vi "ScheduledCmdWindow.vi"(7 "Name (\"\" to Use UUID)":string="Event CSM") -> ()   [LabVIEW 2020, in "CSM-ScheduledCmdWindow.lvlib"]
uses:
  CSM-ScheduledCmdWindow.lvlib
  _support/Command Timer Item.ctl
  <userlib>/_Hooovahh/Array VIMs/Controls/Enum - Order Ascending Descending.ctl
  54d86923-07a1-4d7a-a70d-45b0863b869b.vi
  fe2ecfb7-eb08-4f89-820d-2b95152fbf7e.vi
  dd2ac68a-60a3-4251-9735-56811cc0631c.vi
  96b01cc3-4e05-4812-bc78-c919a57353e8.vi
  <userlib>/_NEVSTOP/Communicable State Machine(CSM)/_Support/GlobalEvent/GEvt-Generate with Rule Check.vi
  <userlib>/_NEVSTOP/Communicable State Machine(CSM)/_Support/GlobalEvent/Cache-GEvt Refs.vi
  <userlib>/_NEVSTOP/Communicable State Machine(CSM)/AdvanceAPI/CSM - Revert Arguments-Safe String.vi
  <userlib>/_NEVSTOP/Communicable State Machine(CSM)/_Shared/Trim Single-line Text.vi
  <userlib>/_NEVSTOP/Communicable State Machine(CSM)/AdvanceAPI/CSM - Make String Arguments Safe.vi
  <userlib>/_NEVSTOP/Communicable State Machine(CSM)/AdvanceAPI/CSM - Break Down Multiple States String.vi
  <userlib>/_NEVSTOP/Communicable State Machine(CSM)/_Support/ChangeFlag/FlagInstance-GEvt Refs.vi
  <userlib>/_NEVSTOP/Communicable State Machine(CSM)/AdvanceAPI/CSM - Keywords.vi
  <userlib>/_NEVSTOP/Communicable State Machine(CSM)/_Support/ChangeFlag/ChangeFlag-Read.vi
  <userlib>/_NEVSTOP/Communicable State Machine(CSM)/AdvanceAPI/CSM - List Modules.vi
  <userlib>/_NEVSTOP/Communicable State Machine(CSM)/_Support/ChangeFlag/ChangeFlagDB.vi
  <userlib>/_NEVSTOP/Communicable State Machine(CSM)/_Support/GlobalEvent/FGV-GlobalEventRef(lvlibp).vi
  <userlib>/_NEVSTOP/Communicable State Machine(CSM)/_Support/GlobalEvent/FGV-GlobalEventQueues(lvlibp).vi
  <userlib>/_NEVSTOP/Communicable State Machine(CSM)/_Support/GlobalEvent/GEvt-Valid Subscribers.vi
  <userlib>/_NEVSTOP/Communicable State Machine(CSM)/_Support/GlobalEvent/LogFilter/LogFilter - Check.vi
  <userlib>/NEVSTOP-Programming-Palette/Dialog & Interface/_support/Autosize All MultiListbox Columns (Uniform Text)_nevstop.vi
  <userlib>/NEVSTOP-Programming-Palette/Dialog & Interface/Fit VI window to Largest Dec_nevstop.vi
  _support/Select Timestamp Dialog.vi
  <userlib>/NEVSTOP-Programming-Palette/Dialog & Interface/Fit VI window to Caller Center_nevstop.vi
  <userlib>/_NEVSTOP/Communicable State Machine(CSM)/addons/API-String-Arugments-Support/_Support/Data To API String Arguments.vi
  <userlib>/_NEVSTOP/Communicable State Machine(CSM)/_Polymophic/Add State(s) to Queue By BOOL(Element).vi
  <userlib>/_NEVSTOP/Communicable State Machine(CSM)/addons/API-String-Arugments-Support/_Support/Convert API String Arguments to Data(variant).vi
  <userlib>/_NEVSTOP/Communicable State Machine(CSM)/_Support/GlobalEvent/LogFilter/LogFilter.lvclass
  <userlib>/_NEVSTOP/Communicable State Machine(CSM)/Communicable State Machine.lvlib
panel:
  out "SharedData":T1[](array[typedef])
  in  "Multicolumn Listbox":i32[](listbox) caption="Table Control"
  in  "Remove Btn":bool
  in  "Add Btn":bool
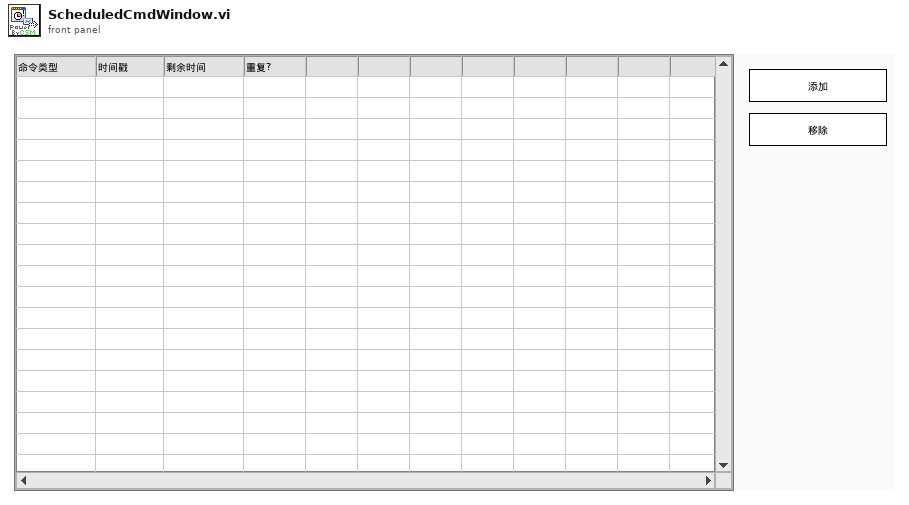
[diagram p1: front panel]
types:
  T1 = typedef "CSM-ScheduledCmdWindow.lvlib/Command Timer Item.ctl" = cluster{"Command":string, "TimeStamp":timestamp, "Daily?":bool}
  T2 = enum32{"Invalid", "Standard", "Closed", "Hidden", "Minimized", "Maximized"}
  T3 = enum32{"invalid app kind", "Development System", "Run Time System", "Student Edition", "Embedded LabVIEW", "Evaluation", "Custom"}
  T4 = typedef "Enum - Order Ascending Descending.ctl" = enum16{"Ascending", "Descending"}
  T5 = typedef "Communicable State Machine.lvlib/_CSM_Response Source Message.ctl" = cluster{"‘State":string, "’Arguments":string, "’Error":errorcluster}
  T6 = cluster{"Current VI Reference":refnum<vi>, "Close Panel on Exit?":bool}
  T7 = cluster{"Core":cluster{"Current VI Reference":refnum<vi>, "Close Panel on Exit?":bool}, "Your Boolean data":bool, "Your string data":string}
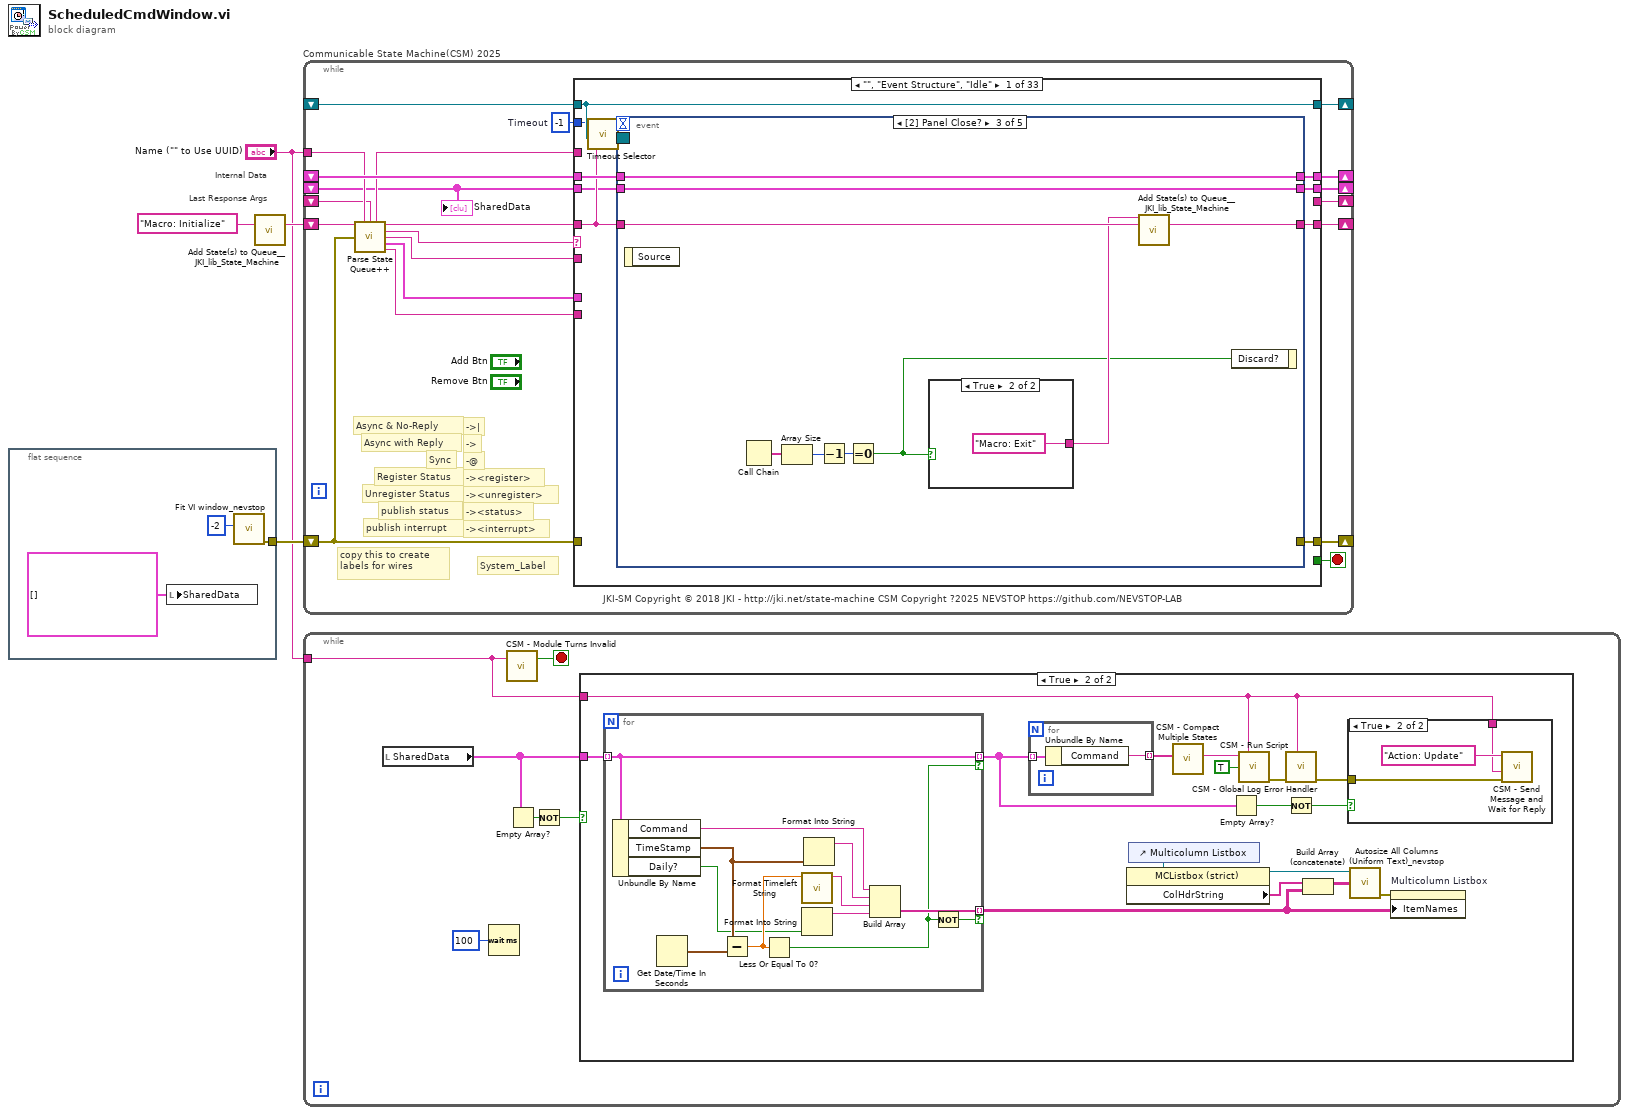
[diagram p0: block diagram]
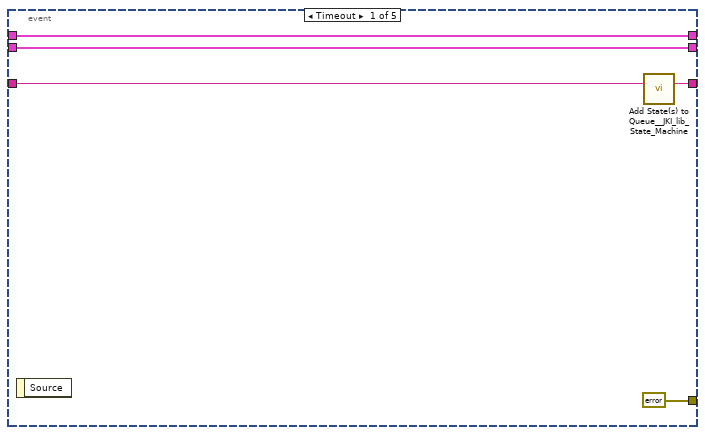
[diagram p2: hidden frame]
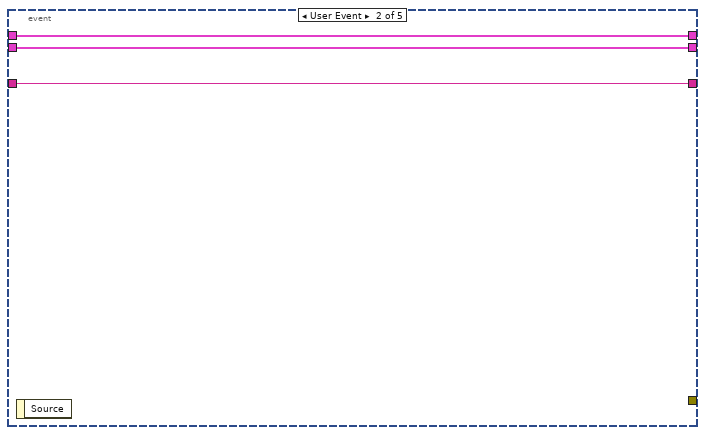
[diagram p3: hidden frame]
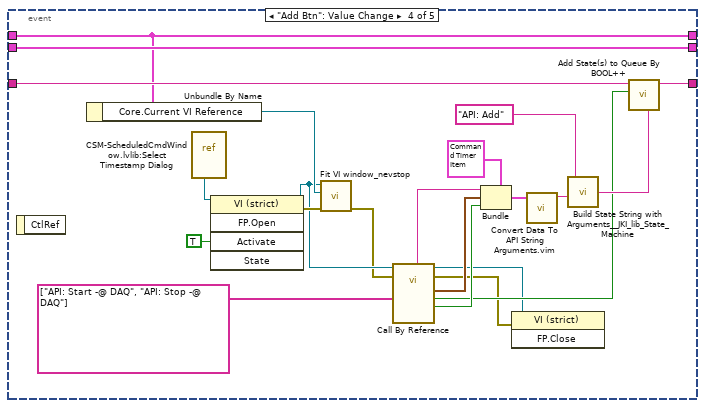
[diagram p5: hidden frame]
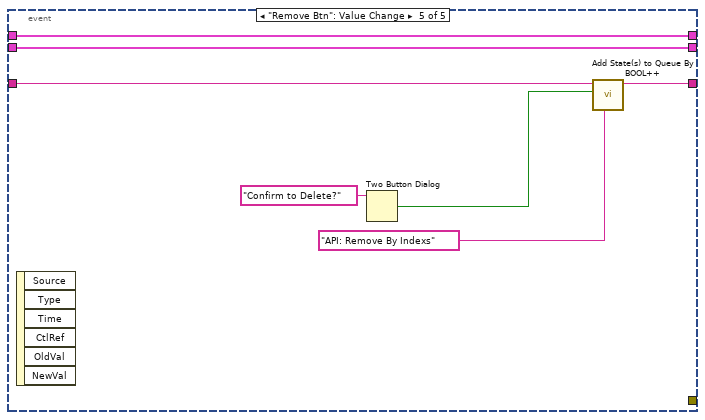
[diagram p6: hidden frame]
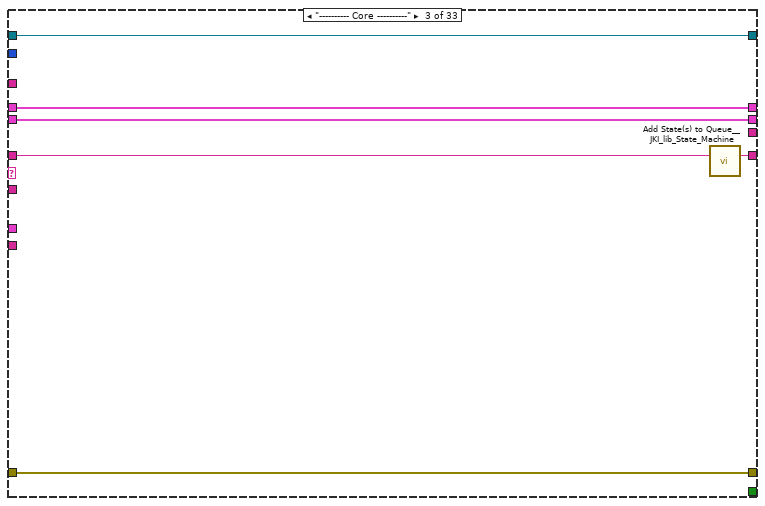
[diagram p8: hidden frame]
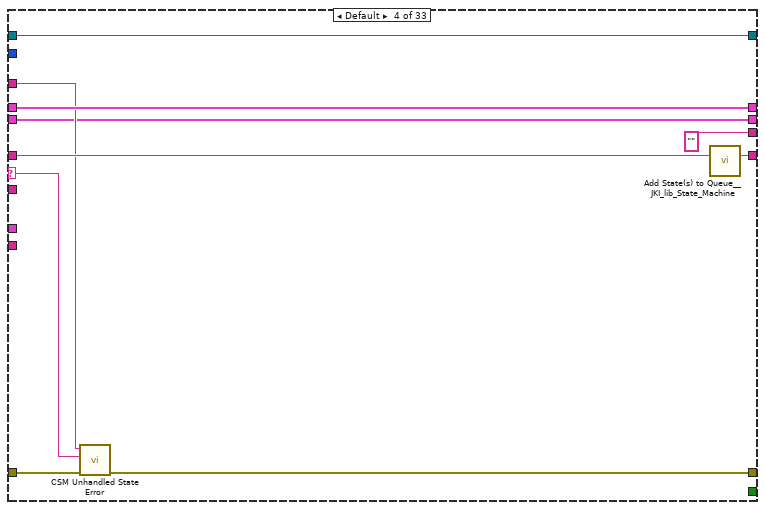
[diagram p9: hidden frame]
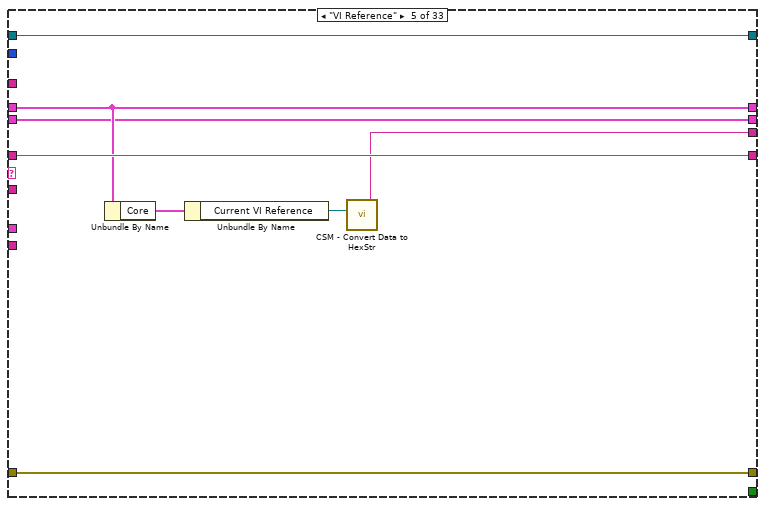
[diagram p10: hidden frame]
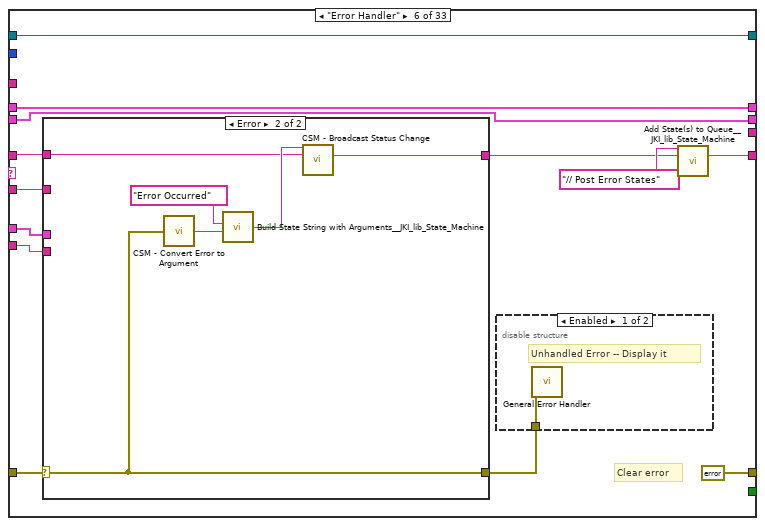
[diagram p11: hidden frame]
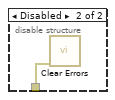
[diagram p12: hidden frame]
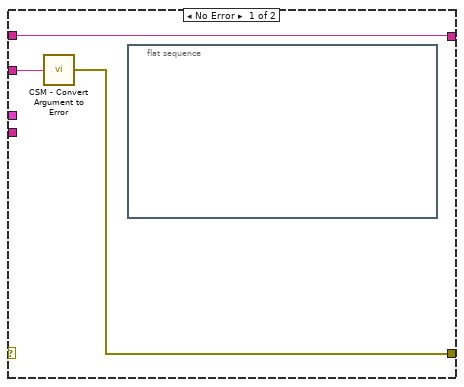
[diagram p13: hidden frame]
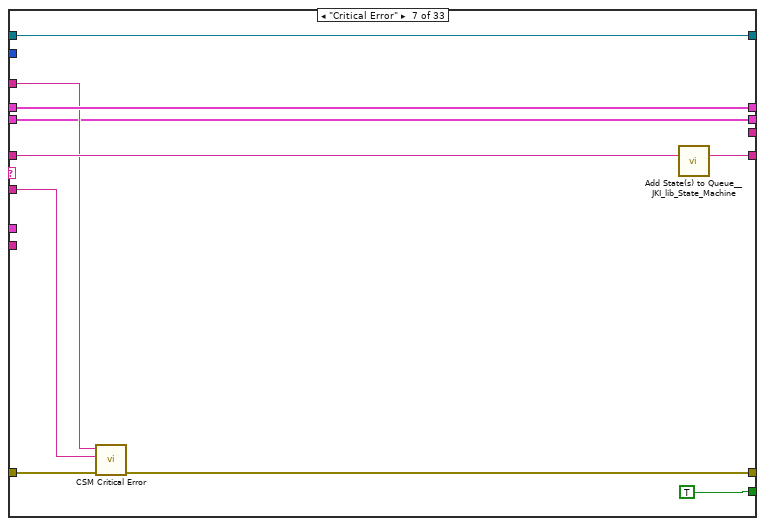
[diagram p14: hidden frame]
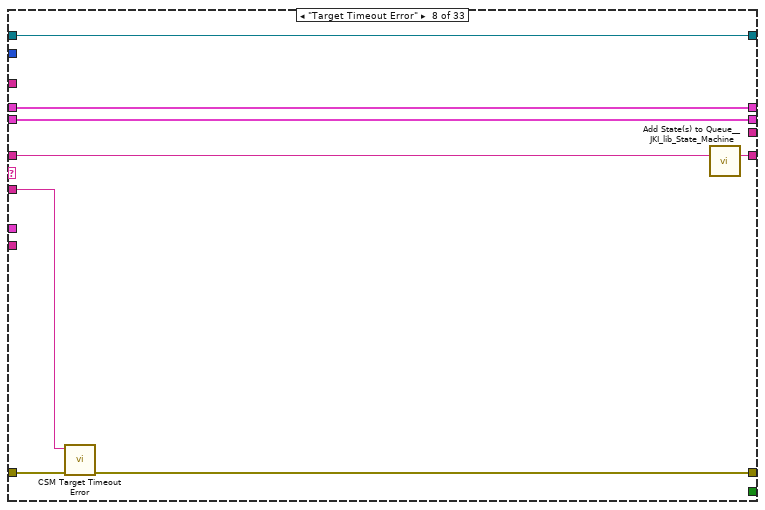
[diagram p15: hidden frame]
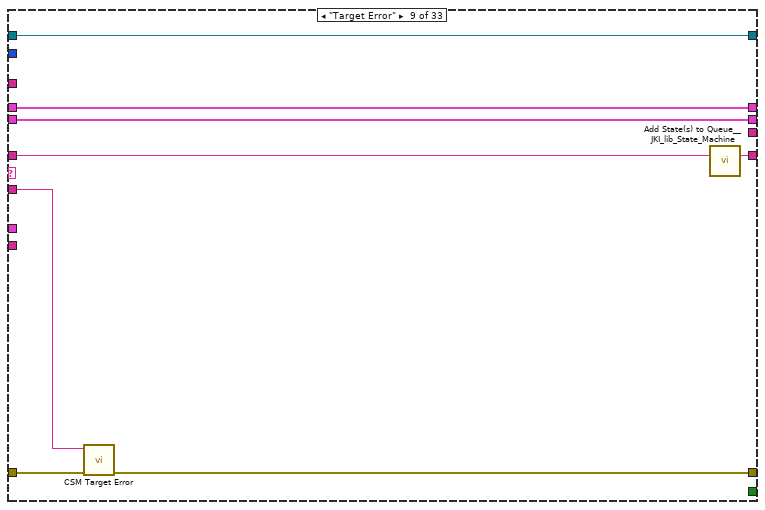
[diagram p16: hidden frame]
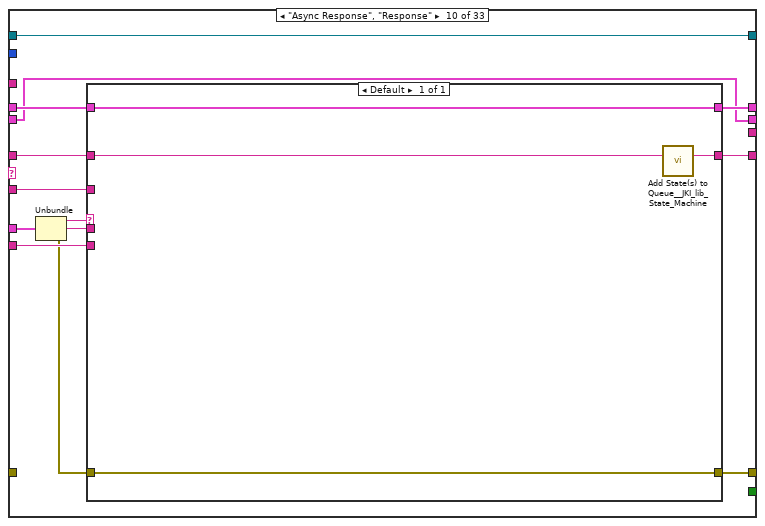
[diagram p17: hidden frame]
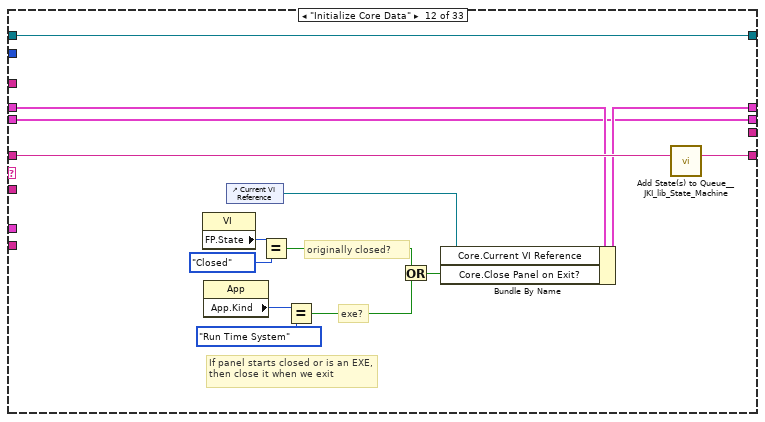
[diagram p19: hidden frame]
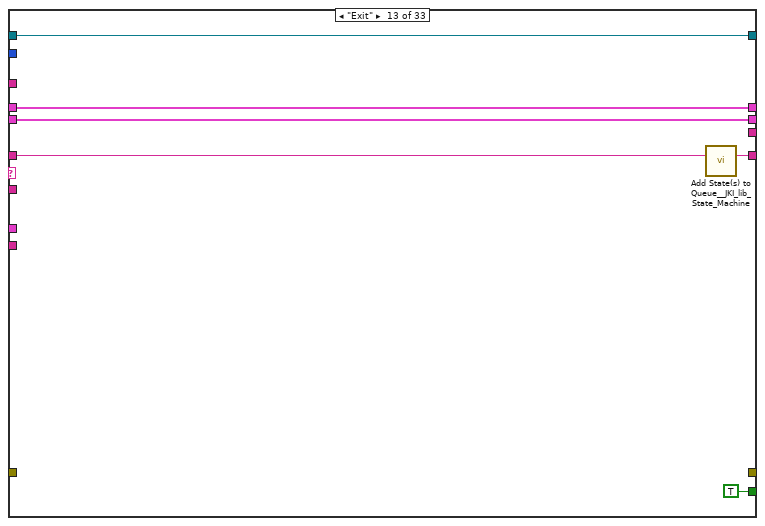
[diagram p20: hidden frame]
diagram:
  # "Last Response Args"
  # "Internal Data"
  n1 = flat-sequence {
    tunnel: [w6] -> w2
    frame #0 {
      n2 = local write "SharedData"(T1[] [] ("SharedData")) -> ()
      n3 = call-poly <userlib>:"Fit VI window_nevstop.vi"("border spacing (2 px)"=-2) -> ("error out"=w6:errorcluster)  [unwired: 5 in, 1 out]
    }
  }
  n4 = call <vilib>:"Add State(s) to Queue__JKI_lib_State_Machine.vi"("State(s) in (\"\")"="Macro: Initialize" ("Init State(\"Macro: Initialize\")")) -> ("States Out"=w3:string)  [unwired: 14 in]
  n5 = while "Communicable State Machine(CSM) 2025" {
    shift-right: [w23] -> _
    shift-left: _ -> [w22]
    shift-right: [w26] -> _
    shift-left: w2 -> [w20]
    shift-right: [w25] -> _
    shift-left: w3 -> [w27]
    tunnel: "Name (\"\" to Use UUID)" -> [w16]
    shift-right: [w19] -> _
    shift-left: _ -> [w11]
    shift-right: [w18] -> _
    shift-left: _ -> [w17]
    shift-right: [w9] -> _
    shift-left: _ -> [w8]
    stop <- w24 stop-if-true
    w21 = -1  # Timeout
    # "-><interrupt>"
    # "-><status>"
    # "-><unregister>"
    # "-><register>"
    # "-@"
    # "->"
    # "->|"
    # "publish interrupt"
    # "publish status"
    # "Unregister Status"
    # "Register Status"
    # "Sync"
    # "Async with Reply"
    # "Async & No-Reply"
    # "copy this to create labels for wires"
    # "System_Label"
    # "JKI-SM Copyright © 2018 JKI - http://jki.net/state-machine CSM Copyright ?2025 NEVSTOP https://github.com/NEVSTOP-LAB"
    n6 = call <userlib>:"Parse State Queue++.vi"("State Queue"=w27, "Name (\"\" to Use UUID)"=w16, "Response Arguments"=w11, "Previous Error"=w20) -> ("Name Used"=w12:string, "Remaining States"=w28:string, "Current State"=w15:string, "Arguments"=w10:string, "Additional Information"=w14:T5, "Source CSM"=w13:string)  [unwired: 6 in]
    n7 = case shown="\"\", \"Event Structure\", \"Idle\"" w15 {
      selector: w15 -> [_ _ _ w99 _ _ _ _ _ _ _ _ _ _ _ _ _ _ _ _ _ _ _ _ _ _ _ _ _ _ _ _ _]
      tunnel: w28 -> [w31 w89 w95 w105 w112 w119 w146 w155 w163 w174 w184 w198 w204 w209 w217 w221 w229 w234 w242 w247 w252 w263 w270 w282 w347 w353 w365 w369 w380 w393 w401 w408 w429]
      tunnel: w10 -> [_ _ _ _ _ w117 w142 w150 w159 w168 _ _ _ _ _ _ _ _ _ _ _ _ w266 w277 _ _ _ _ w373 w386 _ _ _]
      tunnel: w22 -> [w37 w88 w92 w103 w111 w125 w147 w153 w161 w172 w183 w192 w202 w207 _ w220 w225 w232 w241 w246 w250 w261 w268 w279 w345 w351 w363 w368 w379 w392 w399 w406 w427]
      tunnel: [w36 _ w93 w97 w113 errorcluster {"status"=FALSE, "code"=0, "source"=""} ("error out") w139 w149 w157 w171 _ _ _ _ _ w222 w226 _ w236 w245 _ _ w267 w280 _ _ _ _ w371 w383 _ _ _] -> w26
      tunnel: w20 -> [_ _ w93 w98 w113 w123 w140 w151 w158 _ _ _ _ _ _ w222 _ _ _ _ _ _ _ _ _ _ _ _ _ _ _ _ _]
      tunnel: [w38 w89 w94 w104 w112 w121 w145 w154 w162 w175 w184 w197 w203 w208 w216 w221 w228 w233 w242 w247 w251 w262 w269 w281 w346 w352 w364 w369 w380 w393 w400 w407 w428] -> w25
      tunnel: [_ _ _ _ _ _ TRUE _ _ _ _ _ TRUE _ _ _ _ _ _ _ _ _ _ _ _ _ _ _ _ _ _ _ _] -> w24
      tunnel: [w35 w88 w92 w103 w111 w125 w147 w153 w161 w173 w183 w196 w202 w207 w215 w220 w225 w232 w241 w246 w250 w261 w268 w279 w345 w351 w363 w368 w379 w392 w399 w406 w427] -> w23
      tunnel: w21 -> [w33 _ _ _ _ _ _ _ _ _ _ _ _ _ _ _ _ _ _ _ _ _ _ _ _ _ _ _ _ _ _ _ _]
      tunnel: w13 -> [_ _ _ _ _ w116 _ _ _ w169 _ _ _ _ _ _ _ _ _ _ _ _ _ _ _ _ _ _ _ _ _ _ _]
      tunnel: w14 -> [_ _ _ _ _ w115 _ _ _ w170 _ _ _ _ _ _ _ _ _ _ _ _ _ _ _ _ _ _ _ _ _ _ _]
      tunnel: [_ _ _ "" w107 _ _ _ _ _ _ _ _ _ _ _ _ _ _ _ _ _ _ _ _ _ _ _ _ _ _ _ _] -> w19
      tunnel: [w34 w87 w91 w101 w110 w124 w143 w152 w160 w176 w182 w186 w200 w206 w211 w219 w224 w231 w240 w244 w249 w260 w265 w276 w344 w349 w356 w367 w378 w391 w398 w405 w426] -> w18
      tunnel: w17 -> [w34 w87 w91 w101 w110 w124 w143 w152 w160 w176 w182 w186 w200 w206 w211 w219 w224 w231 _ w244 w249 w260 w265 w276 w344 w349 w356 w367 w378 w391 w398 w405 w426]
      tunnel: w12 -> [_ _ _ w100 _ _ w141 _ _ _ _ _ _ _ _ _ _ _ w239 _ _ _ _ _ _ _ _ _ _ _ _ _ _]
      tunnel: [w29 w86 w90 w96 w106 w114 w138 w148 w156 w164 w181 w185 w199 w205 T1[] [] w218 w223 w230 w235 w243 w248 w259 w264 w275 w343 w348 w354 w366 w375 w389 w397 w402 w425] -> w9
      tunnel: w8 -> [w30 w86 w90 w96 w106 w114 w138 w148 w156 w164 w181 w185 w199 w205 _ w218 w223 w230 w235 w243 w248 w259 w264 w275 w343 w348 w354 w366 w376 w390 w397 w404 w425]
      frame "", "Event Structure", "Idle" {
        n8 = call <userlib>:"Timeout Selector.vi"("Remaining States"=w31, "Timeout Expected"=w33) -> ("Timeout"=w32:i32)  [unwired: 5 in]
        n9 = event shown="[2] Panel Close?" {
          selector: w34 -> [_ _ _ _ _]
          dyn-events: _ -> [_ _ _ _ _]
          timeout: w32 -> [_ _ _ _ _]
          tunnel: w31 -> [w43 w45 w55 w72 w82]
          tunnel: [w42 w45 w54 w73 w83] -> w38
          tunnel: w37 -> [w41 w46 w53 w68 w85]
          tunnel: [errorcluster {"status"=FALSE, "code"=0, "source"=""} ("error out") _ _ _ _] -> w36
          tunnel: [w41 w46 w53 w68 w85] -> w35
          tunnel: w30 -> [w39 w44 w52 w78 w84]
          tunnel: [w39 w44 w52 w78 w84] -> w29
          event Timeout {
            n10 = event-data() -> ()  [unwired: 1 in, 1 out]
            n11 = call <vilib>:"Add State(s) to Queue__JKI_lib_State_Machine.vi"("State(s) in (\"\")"=w43) -> ("States Out"=w42:string)  [unwired: 14 in]
          }
          event User Event {
            n12 = event-data() -> ()  [unwired: 1 in, 1 out]
          }
          event Panel Close? {
            n13 = event-data() -> ()  [unwired: 1 in, 1 out]
            n14 = Call Chain() -> (call chain=w47:string[])
            n15 = Array Size(array=w47) -> (size(s)=w48:i32)
            n16 = Decrement(x=w48) -> (x-1=w49:i32)
            n17 = Equal To 0?(x=w49) -> (x = 0?=w50:bool)
            n18 = case shown="True" w50 {
              tunnel: [_ "Macro: Exit"] -> w51
              frame False {
              }
              frame True {
              }
            }
            n19 = call <vilib>:"Add State(s) to Queue__JKI_lib_State_Machine.vi"("State(s) in Front (\"\")"=w51, "State(s) in (\"\")"=w55) -> ("States Out"=w54:string)  [unwired: 13 in]
            n20 = event-data("Discard?"=w50) -> ()  [unwired: 1 in, 1 out]
          }
          event "Add Btn": Value Change {
            n21 = event-data() -> ()  [unwired: 1 in, 1 out]
            n22 = Unbundle By Name(w68) -> ("Core.Current VI Reference"=w67:refnum<vi>)
            n23 = vi-ref "CSM-ScheduledCmdWindow.lvlib:Select Timestamp Dialog.vi"() -> (w70:refnum<vi>)
            n24 = invoke class="VI (strict)" method="FP.Open"(reference=w70, "Activate"=TRUE ("Activate?")) -> (reference out=w66:refnum<vi>, error out=w69:errorcluster)  [unwired: 3 in, 3 out]
            n25 = call-poly <userlib>:"Fit VI window_nevstop.vi"("Error In"=w69, "Background VI Ref (Callee's Caller)"=w67, "VI Ref (calling VI)"=w66) -> ("Error Out"=w60:errorcluster)  [unwired: 3 in, 1 out]
            n26 = call-by-ref "?"(reference=w66, error in=w60, "Command List"=string[] ["API: Start -@ DAQ", "API: Stop -@ DAQ"]) -> (reference out=w58:refnum<vi>, error out=w57:errorcluster, "Daily?"=w64:bool, "Cancelled?"=w63:bool, "Time Stamp out"=w61:timestamp, "Command out"=w62:string)  [unwired: 6 in, 1 out]
            n27 = Bundle(cluster=T1 {"Command"="", "TimeStamp"=timestamp(0 s since 1904-01-01), "Daily?"=FALSE} ("Cluster"), "Command"=w62, "TimeStamp"=w61, "Daily?"=w64) -> (w76:T1)
            n28 = invoke class="VI (strict)" method="FP.Close"(reference=w58, error in=w57) -> ()  [unwired: 1 in, 3 out]
            n29 = call "Convert Data To API String Arguments.vim"("Data"=w76) -> ("API String"=w75:string)  [unwired: 7 in, 1 out]
            n30 = call <vilib>:"Build State String with Arguments__JKI_lib_State_Machine.vi"("Arguments (\"\")"=w75, "State"="API: Add") -> ("State with Arguments"=w71:string)  [unwired: 4 in]
            n31 = call-poly <userlib>:"Add State(s) to Queue By BOOL++.vi"("FALSE (\"\")"=w71, "Condition"=w63, "State Queue (\"\")"=w72) -> ("Remaining States"=w73:string)  [unwired: 8 in]
          }
          event "Remove Btn": Value Change {
            n32 = event-data() -> ()  [unwired: 1 in, 6 out]
            n33 = Two Button Dialog(message="Confirm to Delete?") -> (T button?=w80:bool)  [unwired: 2 in]
            n34 = call-poly <userlib>:"Add State(s) to Queue By BOOL++.vi"("TRUE (\"\")"="API: Remove By Indexs" ("TRUE (\"\")"), "Condition"=w80, "State Queue (\"\")"=w82) -> ("Remaining States"=w83:string)  [unwired: 8 in]
          }
        }
      }
      frame "CSM Documentation" {
      }
      frame "---------- Core ----------" {
        n35 = call <vilib>:"Add State(s) to Queue__JKI_lib_State_Machine.vi"("State(s) in (\"\")"=w95) -> ("States Out"=w94:string)  [unwired: 14 in]
      }
      frame Default {
        n36 = call <userlib>:"CSM Unhandled State Error.vi"("error in (no error)"=w98, "Undefined State"=w99, "CSM Name"=w100) -> ("error out"=w97:errorcluster)  [unwired: 8 in]
        n37 = call <vilib>:"Add State(s) to Queue__JKI_lib_State_Machine.vi"("State(s) in (\"\")"=w105) -> ("States Out"=w104:string)  [unwired: 14 in]
      }
      frame "VI Reference" {
        n38 = Unbundle By Name(w111) -> ("Core"=w109:T6)
        n39 = Unbundle By Name(w109) -> ("Current VI Reference"=w108:refnum<vi>)
        n40 = call <userlib>:"CSM - Convert Data to HexStr.vi"("Variant"=w108) -> ("HEX String (0-9,A-F)"=w107:string)  [unwired: 8 in]
      }
      frame "Error Handler" {
        # "Clear error"
        n41 = case shown="Error" w123 {
          selector: w123 -> [_ w132]
          tunnel: [w130 w134] -> w120
          tunnel: w119 -> [w130 w133]
          tunnel: [w129 w132] -> w118
          tunnel: w117 -> [w131 _]
          tunnel: w116 -> [_ _]
          tunnel: w115 -> [_ _]
          frame No Error {
            n42 = call <userlib>:"CSM - Convert Argument to Error.vi"("Argument"=w131) -> ("Error"=w129:errorcluster)  [unwired: 4 in]
            n43 = flat-sequence {
              frame #0 {
              }
            }
          }
          frame Error {
            n44 = call <userlib>:"CSM - Convert Error to Argument.vi"("Error"=w132) -> ("Argument"=w136:string)  [unwired: 4 in]
            n45 = call <vilib>:"Build State String with Arguments__JKI_lib_State_Machine.vi"("Arguments (\"\")"=w136, "State"="Error Occurred" ("Status with Arguments")) -> ("State with Arguments"=w135:string)  [unwired: 4 in]
            n46 = call <userlib>:"CSM - Broadcast Status Change.vi"("Status With Arguments"=w135, "State Queue"=w133) -> ("Remaining States"=w134:string)  [unwired: 13 in]
          }
        }
        n47 = disable-structure shown="Enabled" {
          disable-tunnel: w118 -> [w127 w128]
          frame Enabled {
            # "Unhandled Error -- Display it"
            n48 = call <vilib>:"General Error Handler.vi"("error in (no error)"=w127) -> ()  [unwired: 10 in, 5 out]
          }
          frame Disabled {
            n49 = call <vilib>:"Clear Errors.vi"("error in (no error)"=w128) -> ()  [unwired: 5 in, 2 out]
          }
        }
        n50 = call <vilib>:"Add State(s) to Queue__JKI_lib_State_Machine.vi"("State(s) in Front (\"\")"="// Post Error States", "State(s) in (\"\")"=w120) -> ("States Out"=w121:string)  [unwired: 13 in]
      }
      frame "Critical Error" {
        n51 = call <userlib>:"CSM Critical Error.vi"("error in (no error)"=w140, "Arugments (As Reason)"=w142, "CSM Name"=w141) -> ("error out"=w139:errorcluster)  [unwired: 8 in]
        n52 = call <vilib>:"Add State(s) to Queue__JKI_lib_State_Machine.vi"("State(s) in (\"\")"=w146) -> ("States Out"=w145:string)  [unwired: 14 in]
      }
      frame "Target Timeout Error" {
        n53 = call <userlib>:"CSM Target Timeout Error.vi"("error in (no error)"=w151, "Arguments (As CSM Name)"=w150) -> ("error out"=w149:errorcluster)  [unwired: 9 in]
        n54 = call <vilib>:"Add State(s) to Queue__JKI_lib_State_Machine.vi"("State(s) in (\"\")"=w155) -> ("States Out"=w154:string)  [unwired: 14 in]
      }
      frame "Target Error" {
        n55 = call <userlib>:"CSM Target Error.vi"("error in (no error)"=w158, "Arguments (As CSM Name)"=w159) -> ("error out"=w157:errorcluster)  [unwired: 9 in]
        n56 = call <vilib>:"Add State(s) to Queue__JKI_lib_State_Machine.vi"("State(s) in (\"\")"=w163) -> ("States Out"=w162:string)  [unwired: 14 in]
      }
      frame "Async Response", "Response" {
        n57 = Unbundle(w170) -> ("‘State"=w167:string, "’Arguments"=w166:string, "’Error"=w165:errorcluster)
        n58 = case shown="Default" w167 {
          tunnel: [w177] -> w175
          tunnel: w174 -> [w178]
          tunnel: [w180] -> w173
          tunnel: w172 -> [w180]
          tunnel: [w179] -> w171
          tunnel: w165 -> [w179]
          tunnel: w169 -> [_]
          tunnel: w168 -> [_]
          tunnel: w166 -> [_]
          frame Default {
            n59 = call <vilib>:"Add State(s) to Queue__JKI_lib_State_Machine.vi"("State(s) in (\"\")"=w178) -> ("States Out"=w177:string)  [unwired: 14 in]
          }
        }
      }
      frame "Async Message Posted" {
      }
      frame "Initialize Core Data" {
        # "originally closed?"
        # "exe?"
        # "If panel starts closed or is an EXE, then close it when we exit"
        n60 = property class="VI"() -> ("FP.State"=w189:T2)  [unwired: 2 in, 2 out]
        n61 = property class="App"() -> ("App.Kind"=w195:T3)  [unwired: 2 in, 2 out]
        n62 = control-ref of="Current VI Reference"() -> (w190:refnum<vi>)
        n63 = Equal?(x=w189, y=T2."Closed" ("Front Panel Window:State")) -> (x = y?=w187:bool)
        n64 = Equal?(x=w195, y=T3."Run Time System" ("Application:Kind")) -> (x = y?=w193:bool)
        n65 = Or(x=w187, y=w193) -> (x .or. y?=w191:bool)
        n66 = Bundle By Name(cluster=w192, "Core.Current VI Reference"=w190, "Core.Close Panel on Exit?"=w191) -> (w196:T7)
        n67 = call <vilib>:"Add State(s) to Queue__JKI_lib_State_Machine.vi"("State(s) in (\"\")"=w198) -> ("States Out"=w197:string)  [unwired: 14 in]
      }
      frame "Exit" {
        n68 = call <vilib>:"Add State(s) to Queue__JKI_lib_State_Machine.vi"("State(s) in (\"\")"=w204) -> ("States Out"=w203:string)  [unwired: 14 in]
      }
      frame "---------- Data ----------" {
        n69 = call <vilib>:"Add State(s) to Queue__JKI_lib_State_Machine.vi"("State(s) in (\"\")"=w209) -> ("States Out"=w208:string)  [unwired: 14 in]
      }
      frame "Data: Initialize" {
        w212 = T6 {"Current VI Reference"=refnum, "Close Panel on Exit?"=FALSE}  # Core
        w214 = TRUE  # Your Boolean data
        w213 = ""  # Your string data
        n70 = call <vilib>:"Add State(s) to Queue__JKI_lib_State_Machine.vi"("State(s) in (\"\")"=w217) -> ("States Out"=w216:string)  [unwired: 14 in]
        n71 = Bundle("Core"=w212, "Your Boolean data"=w214, "Your string data"=w213) -> (w215:T7)  [unwired: 1 in]
      }
      frame "Data: Load Configurations" {
      }
      frame "Data: Cleanup" {
        n72 = Unbundle By Name(w225) -> ("Core.Current VI Reference"=w227:refnum<vi>)
        n73 = Close Reference(reference=w227) -> (error out=w226:errorcluster)  [unwired: 1 in]
        n74 = call <vilib>:"Add State(s) to Queue__JKI_lib_State_Machine.vi"("State(s) in (\"\")"=w229) -> ("States Out"=w228:string)  [unwired: 14 in]
      }
      frame "---------- Events ----------" {
        n75 = call <vilib>:"Add State(s) to Queue__JKI_lib_State_Machine.vi"("State(s) in (\"\")"=w234) -> ("States Out"=w233:string)  [unwired: 14 in]
      }
      frame "Events: Register" {
        n76 = call <userlib>:"CSM - Get New State Notifier Event.vi"("Name (\"\" to Use UUID)"=w239) -> ("error out"=w237:errorcluster, "New State Notifier Event"=w238:refnum<user-event>)  [unwired: 9 in]
        n77 = register-events(error in=w237, w238) -> (reference out=w240:refnum<event-registration>, error out=w236:errorcluster)  [unwired: 1 in]
      }
      frame "Events: Unregister" {
        n78 = Unregister For Events(event registration refnum=w244) -> (error out=w245:errorcluster)  [unwired: 1 in]
      }
      frame "---------- UI ----------" {
        n79 = call <vilib>:"Add State(s) to Queue__JKI_lib_State_Machine.vi"("State(s) in (\"\")"=w252) -> ("States Out"=w251:string)  [unwired: 14 in]
      }
      frame "UI: Initialize" {
        w253 = string[][] [] ("Item Names")
        n80 = control-ref of="Multicolumn Listbox"() -> (w255:refnum<vi>)
        n81 = property class="MCListbox (strict)"(reference=w255) -> (reference out=w256:refnum<vi>, "ColHdrString"=w257:string[])  [unwired: 1 in, 1 out]
        n82 = Build Array (concatenate)(w257, w253) -> (w258:string[][])
        n83 = call-poly <userlib>:"Autosize All Columns (Uniform Text)_nevstop.vi"("Array"=w258, "Control in"=w256) -> ("error out"=w254:errorcluster)  [unwired: 8 in, 1 out]
        n84 = property on="Multicolumn Listbox" class="MCListbox (strict)"(error in=w254, "ItemNames"=w253) -> ()  [unwired: 1 in, 2 out]
        n85 = call <vilib>:"Add State(s) to Queue__JKI_lib_State_Machine.vi"("State(s) in (\"\")"=w263) -> ("States Out"=w262:string)  [unwired: 14 in]
      }
      frame "UI: Cursor Set" {
        # "Argument"
        n86 = disable-structure shown="TARGET_TYPE!=Windows" {
          disable-tunnel: [w272 _] -> w267
          disable-tunnel: w266 -> [w271 _]
          frame condition #0 (active) {
            n87 = case shown="\"Idle\", Default" w271 {
              tunnel: [w273 w274] -> w272
              frame "Idle", Default {
                n88 = call <vilib>:"Unset Busy.vi"() -> ("error out"=w273:errorcluster)  [unwired: 11 in]
              }
              frame "Busy" {
                n89 = call <vilib>:"Set Busy.vi"() -> ("error out"=w274:errorcluster)  [unwired: 10 in, 1 out]
              }
            }
          }
          frame condition #1 {
          }
        }
        n90 = call <vilib>:"Add State(s) to Queue__JKI_lib_State_Machine.vi"("State(s) in (\"\")"=w270) -> ("States Out"=w269:string)  [unwired: 14 in]
      }
      frame "UI: Front Panel State" {
        # "Argument"
        n91 = Unbundle By Name(w279) -> ("Core.Current VI Reference"=w278:refnum<vi>)
        n92 = case shown="\"Minimize\", \"Minimized\"" w277 {
          tunnel: [w289 w302 w313 w325 w337] -> w280
          tunnel: w278 -> [w288 w300 w312 w324 w336]
          frame "Open", "Standard", Default {
            w283 = T2."Standard" ("State")
            n93 = property class="VI"(reference=w288) -> (reference out=w286:refnum<vi>, error out=w287:errorcluster, "FP.State"=w285:T2)  [unwired: 1 in]
            n94 = Not Equal?(x=w285, y=w283) -> (x != y?=w284:bool)
            n95 = case shown="True" w284 {
              tunnel: [w293 w295] -> w289
              tunnel: w287 -> [w292 w295]
              tunnel: w286 -> [w291 _]
              tunnel: w283 -> [w290 _]
              frame True {
                n96 = invoke class="VI" method="FP.Open"(reference=w291, error in=w292, "Activate"=TRUE, "State"=w290) -> (error out=w293:errorcluster)  [unwired: 1 in, 4 out]
              }
              frame False {
              }
            }
          }
          frame "Close", "Closed" {
            n97 = property class="VI"(reference=w300) -> (reference out=w299:refnum<vi>, error out=w301:errorcluster, "FP.State"=w297:T2)  [unwired: 1 in]
            n98 = Not Equal?(x=w297, y=T2."Closed" ("Front Panel Window:State")) -> (x != y?=w296:bool)
            n99 = case shown="True" w296 {
              tunnel: [w303 w306] -> w302
              tunnel: w301 -> [w303 w305]
              tunnel: w299 -> [_ w304]
              frame False {
              }
              frame True {
                n100 = invoke class="VI" method="FP.Close"(reference=w304, error in=w305) -> (error out=w306:errorcluster)  [unwired: 1 in, 2 out]
              }
            }
          }
          frame "Hidden", "Hide" {
            w307 = T2."Hidden" ("State")
            n101 = property class="VI"(reference=w312) -> (reference out=w310:refnum<vi>, error out=w311:errorcluster, "FP.State"=w309:T2)  [unwired: 1 in]
            n102 = Not Equal?(x=w309, y=w307) -> (x != y?=w308:bool)
            n103 = case shown="True" w308 {
              tunnel: [w317 w318] -> w313
              tunnel: w311 -> [w316 w318]
              tunnel: w310 -> [w315 _]
              tunnel: w307 -> [w314 _]
              frame True {
                n104 = invoke class="VI" method="FP.Open"(reference=w315, error in=w316, "State"=w314) -> (error out=w317:errorcluster)  [unwired: 2 in, 4 out]
              }
              frame False {
              }
            }
          }
          frame "Minimize", "Minimized" {
            w319 = T2."Minimized" ("State")
            n105 = property class="VI"(reference=w324) -> (reference out=w322:refnum<vi>, error out=w323:errorcluster, "FP.State"=w321:T2)  [unwired: 1 in]
            n106 = Not Equal?(x=w321, y=w319) -> (x != y?=w320:bool)
            n107 = case shown="False" w320 {
              tunnel: [w329 w330] -> w325
              tunnel: w323 -> [w328 w330]
              tunnel: w322 -> [w327 _]
              tunnel: w319 -> [w326 _]
              frame True {
                n108 = invoke class="VI" method="FP.Open"(reference=w327, error in=w328, "State"=w326) -> (error out=w329:errorcluster)  [unwired: 2 in, 4 out]
              }
              frame False {
              }
            }
          }
          frame "Maximize", "Maximized" {
            w331 = T2."Maximized" ("State")
            n109 = property class="VI"(reference=w336) -> (reference out=w334:refnum<vi>, error out=w335:errorcluster, "FP.State"=w333:T2)  [unwired: 1 in]
            n110 = Not Equal?(x=w333, y=w331) -> (x != y?=w332:bool)
            n111 = case shown="True" w332 {
              tunnel: [w341 w342] -> w337
              tunnel: w335 -> [w340 w342]
              tunnel: w334 -> [w339 _]
              tunnel: w331 -> [w338 _]
              frame True {
                n112 = invoke class="VI" method="FP.Open"(reference=w339, error in=w340, "State"=w338) -> (error out=w341:errorcluster)  [unwired: 2 in, 4 out]
              }
              frame False {
              }
            }
          }
        }
        n113 = call <vilib>:"Add State(s) to Queue__JKI_lib_State_Machine.vi"("State(s) in (\"\")"=w282) -> ("States Out"=w281:string)  [unwired: 14 in]
      }
      frame "---------- Macro ----------" {
        n114 = call <vilib>:"Add State(s) to Queue__JKI_lib_State_Machine.vi"("State(s) in (\"\")"=w347) -> ("States Out"=w346:string)  [unwired: 14 in]
      }
      frame "Macro: Initialize" {
        w350 = "Data: Initialize\nInitialize Core Data\nEvents: Register\nUI: Initialize\n//UI: Front Panel State >> Open"  # Data: Initialize Initialize Core Data Events: Register UI: Initialize //UI: Front Panel State >> Open
        n115 = call <vilib>:"Add State(s) to Queue__JKI_lib_State_Machine.vi"("State(s) in Front (\"\")"=w350, "State(s) in (\"\")"=w353) -> ("States Out"=w352:string)  [unwired: 13 in]
      }
      frame "Macro: Exit" {
        n116 = Unbundle By Name(w363) -> ("Core.Close Panel on Exit?"=w362:bool)
        n117 = Select(t="UI: Front Panel State >> Close", s=w362, f="") -> (s? t:f=w359:string)
        n118 = call <vilib>:"Add State(s) to Queue__JKI_lib_State_Machine.vi"("State(s) in Front (\"\")"="//Exit Sub-Modules ", "State(s) in (\"\")"=w359, "State(s) at Back (\"\")"="Data: Cleanup\nEvents: Unregister\nExit") -> ("States Out"=w357:string)  [unwired: 12 in]
        n119 = call <vilib>:"Add State(s) to Queue__JKI_lib_State_Machine.vi"("State(s) in Front (\"\")"=w357, "State(s) in (\"\")"=w365) -> ("States Out"=w364:string)  [unwired: 13 in]
      }
      frame "---------- API ----------" {
      }
      frame "API: Add" {
        n120 = disable-structure shown="Disabled" {
          disable-tunnel: w376 -> [w382 _]
          disable-tunnel: [w381 _] -> w374
          frame Disabled {
            n121 = Index Array(array=w382) -> (element=w381:T1)  [unwired: 1 in]
          }
          frame Enabled {
          }
        }
        n122 = call "Convert API String Arguments to Data.vim"("Reference Type"=w374, "Strict Label Check? (T)"=TRUE, "API String"=w373) -> ("error out"=w371:errorcluster, "Data"=w372:T1)  [unwired: 5 in]
        n123 = Build Array (concatenate)(w376, w372) -> (w377:T1[])
        n124 = call "Reorder Commands.vi"("Array in"=w377) -> ("Array out"=w375:T1[])  [unwired: 10 in]
      }
      frame "API: Remove By Indexs" {
        n125 = call "Convert API String Arguments to Data.vim"("Reference Type"="Multicolumn Listbox", "API String"=w386) -> ("error out"=w383:errorcluster, "Data"=w384:i32[])  [unwired: 6 in]
        n126 = call "Sort 1D Array-VIM.vim"("Order (Ascending)"=Enum_-_Order_Ascending_Descending."Descending", "Array in"=w384) -> ("Sorted Array out"=w387:i32[])  [unwired: 8 in, 1 out]
        n127 = for "For Each element to delete" {
          tunnel: w387 -> [w396] mode=indexing
          shift-right: [w395] -> w389
          shift-left: w390 -> [w394]
          # "delete element"
          n128 = Delete From Array(array=w394, index=w396) -> (array with subset deleted=w395:T1[])  [unwired: 1 in, 1 out]
        }
      }
      frame "---------- Action ----------" {
        n129 = call <vilib>:"Add State(s) to Queue__JKI_lib_State_Machine.vi"("State(s) in (\"\")"=w401) -> ("States Out"=w400:string)  [unwired: 14 in]
      }
      frame "Action: Update" {
        n130 = for {
          tunnel: w404 -> [w417] mode=indexing
          tunnel: [w420] -> _ mode=indexing if=w412
          tunnel: [w418] -> w403 mode=indexing if=w414
          n131 = Unbundle By Name(w417) -> ("Command"=w409:string, "TimeStamp"=w421:timestamp, "Daily?"=w410:bool)
          n132 = Get Date/Time In Seconds() -> (seconds since 1Jan1904=w423:timestamp)
          n133 = Subtract(x=w421, y=w423) -> (x-y=w424:dbl)
          n134 = Less Or Equal To 0?(x=w424) -> (x <= 0?=w413:bool)
          n135 = Format Into String(w421) -> (resulting string=w419:string)  [unwired: 3 in, 1 out]
          n136 = call "Format Timeleft String.vi"("second"=w424) -> ("Elapsed Time"=w422:string)  [unwired: 10 in]
          n137 = Format Into String(w410) -> (resulting string=w411:string)  [unwired: 3 in, 1 out]
          n138 = Build Array(w409, w419, w422, w411) -> (w420:string[])
          n139 = call "Increase command Date.vi"("Cluster 2"=w417) -> ("Cluster 2"=w416:T1)  [unwired: 10 in]
          n140 = Select(t=w416, s=w413, f=w417) -> (s? t:f=w418:T1)
          n141 = Not(x=w413) -> (.not. x?=w415:bool)
          n142 = Or(x=w415, y=w410) -> (x .or. y?=w414:bool)
          n143 = Not(x=w413) -> (.not. x?=w412:bool)
        }
        n144 = call "Reorder Commands.vi"("Array in"=w403) -> ("Array out"=w402:T1[])  [unwired: 10 in]
        n145 = call <vilib>:"Add State(s) to Queue__JKI_lib_State_Machine.vi"("State(s) in (\"\")"=w408) -> ("States Out"=w407:string)  [unwired: 14 in]
      }
      frame "Action: action2" {
        n146 = call <vilib>:"Add State(s) to Queue__JKI_lib_State_Machine.vi"("State(s) in (\"\")"=w429) -> ("States Out"=w428:string)  [unwired: 14 in]
      }
    }
    "SharedData" <- w8
  }
  n147 = while {
    tunnel: "Name (\"\" to Use UUID)" -> [w430]
    stop <- w434 stop-if-true
    n148 = local read "SharedData"() -> (w432:T1[])
    n149 = Wait (ms)(milliseconds to wait=u32 100) -> ()  [unwired: 1 out]
    n150 = call <userlib>:"CSM - Module Turns Invalid.vi"("CSM Name"=w430) -> ("Turn Invalid (Exit)?"=w434:bool)  [unwired: 2 in]
    n151 = Empty Array?(array=w432) -> (empty?=w435:bool)
    n152 = Not(x=w435) -> (.not. x?=w431:bool)
    n153 = case shown="True" w431 {
      tunnel: w432 -> [_ w451]
      tunnel: w430 -> [_ w439]
      frame False {
        (unwired) FALSE
      }
      frame True {
        n154 = for {
          tunnel: w451 -> [w460] mode=indexing
          tunnel: [w462] -> w450 mode=indexing if=w459
          tunnel: [w460] -> w442 mode=indexing if=w455
          n155 = Unbundle By Name(w460) -> ("Command"=w456:string, "TimeStamp"=w463:timestamp, "Daily?"=w457:bool)
          n156 = Get Date/Time In Seconds() -> (seconds since 1Jan1904=w465:timestamp)
          n157 = Subtract(x=w463, y=w465) -> (x-y=w466:dbl)
          n158 = Less Or Equal To 0?(x=w466) -> (x <= 0?=w455:bool)
          n159 = call "Format Timeleft String.vi"("second"=w466) -> ("Elapsed Time"=w464:string)  [unwired: 10 in]
          n160 = Format Into String(w457) -> (resulting string=w458:string)  [unwired: 3 in, 1 out]
          n161 = Format Into String(w463) -> (resulting string=w461:string)  [unwired: 3 in, 1 out]
          n162 = Build Array(w456, w461, w464, w458) -> (w462:string[])
          n163 = Not(x=w455) -> (.not. x?=w459:bool)
        }
        n164 = for {
          tunnel: w442 -> [w468] mode=indexing
          tunnel: [w467] -> w447 mode=indexing
          n165 = Unbundle By Name(w468) -> ("Command"=w467:string)
        }
        n166 = control-ref of="Multicolumn Listbox"() -> (w448:refnum<vi>)
        n167 = property class="MCListbox (strict)"(reference=w448) -> (reference out=w438:refnum<vi>, "ColHdrString"=w437:string[])  [unwired: 1 in, 1 out]
        n168 = call <userlib>:"CSM - Compact Multiple States.vi"("Multiple States"=w447) -> ("States"=w446:string)  [unwired: 9 in]
        n169 = Empty Array?(array=w442) -> (empty?=w441:bool)
        n170 = call <userlib>:"CSM - Run Script.vi"("CSM Scripts"=w446, "Current Module (\"\" to Generate an ID)"=w439, "Continue If Error? (F)"=TRUE) -> ("error out"=w444:errorcluster)  [unwired: 10 in, 2 out]
        n171 = call <userlib>:"CSM - Global Log Error Handler.vi"("Place (\"\" to Use VI's Name)"=w439, "Error In"=w444) -> ("error out"=w443:errorcluster)  [unwired: 9 in]
        n172 = Not(x=w441) -> (.not. x?=w440:bool)
        n173 = Build Array (concatenate)(w437, w450) -> (w436:string[][])
        n174 = case shown="True" w440 {
          tunnel: w443 -> [_ w454]
          tunnel: w439 -> [_ w452]
          frame False {
          }
          frame True {
            n175 = call <userlib>:"CSM - Send Message and Wait for Reply.vi"("Error In (No Error)"=w454, "Target Module"=w452, "State"="Action: Update") -> ()  [unwired: 6 in, 3 out]
          }
        }
        n176 = call-poly <userlib>:"Autosize All Columns (Uniform Text)_nevstop.vi"("Array"=w436, "Control in"=w438) -> ("error out"=w449:errorcluster)  [unwired: 8 in, 1 out]
        n177 = property on="Multicolumn Listbox" class="MCListbox (strict)"(error in=w449, "ItemNames"=w450) -> ()  [unwired: 1 in, 2 out]
      }
    }
  }
